vi "Parse Any Restric Data.vi"(8 "Error In":errorcluster, 10 "Data":string, 11 "ERD_Always Show in":T1) -> (0 "Error Out":errorcluster, 1 "CSV Data Out":string[](array[string]), 3 "ERD_Always Show out":T1)   [LabVIEW 2023]
uses:
  type defs/ERD_Always_Show_JL.ctl
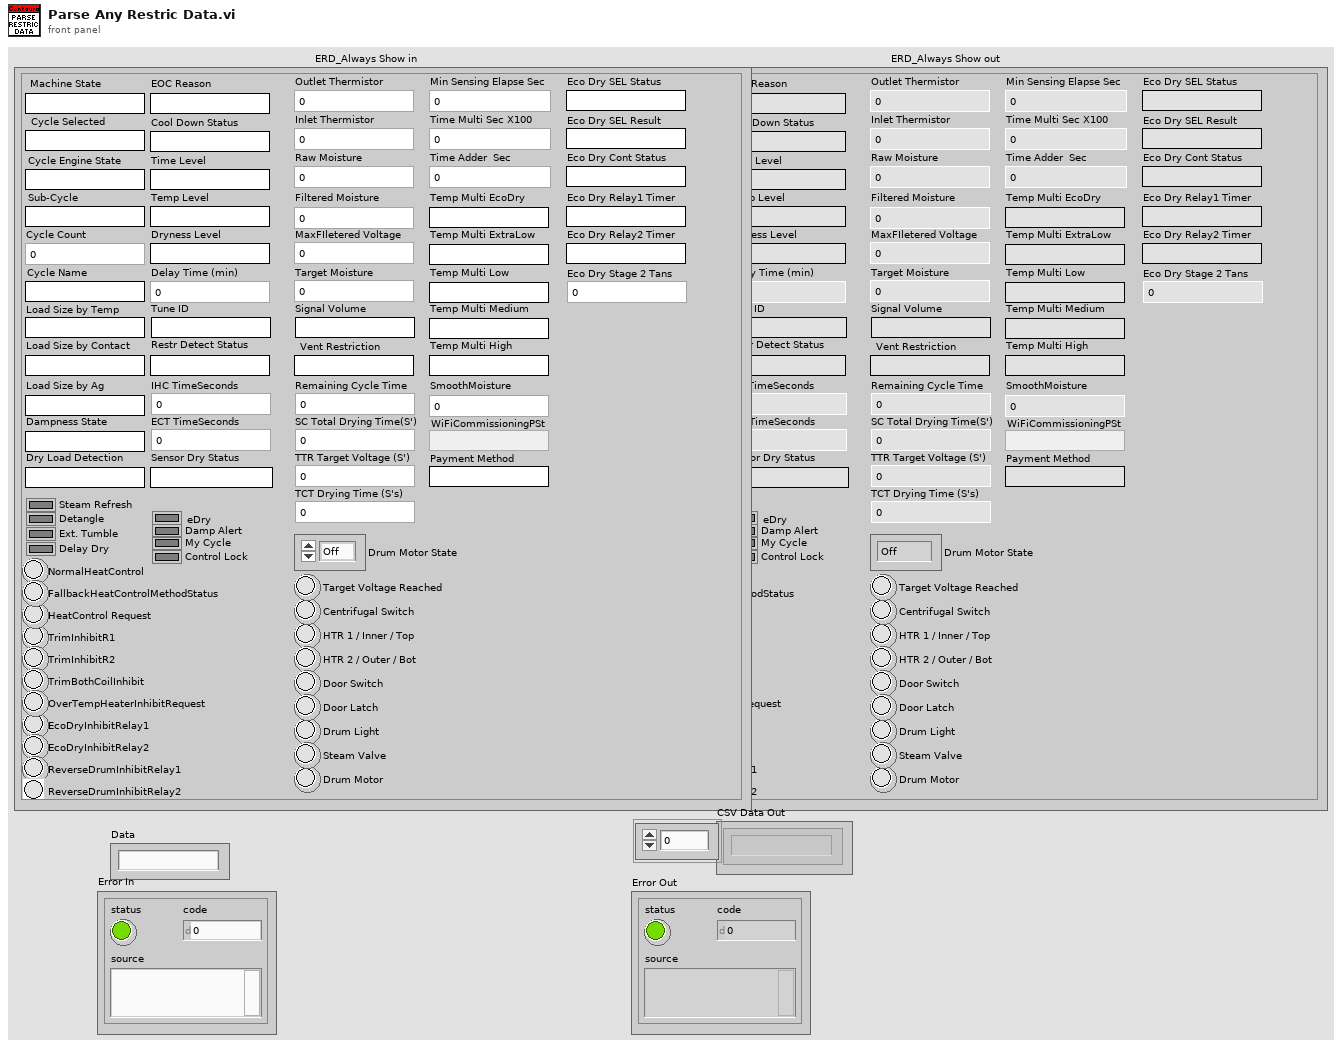
[diagram p1: front panel]
types:
  T1 = typedef "ERD_Always_Show_JL.ctl" = cluster{"Inlet Thermistor":u16, "Machine State":string, "Filtered Moisture":u16, "Cycle Selected":string, "HTR 1 / Inner / Top":bool, "HTR 2 / Outer / Bot":bool, "Door Switch":bool, "Drum Light":bool, "Cycle Engine State":string, "Centrifugal Switch":bool, "Drum Motor":bool, "Cycle Count":u32, "Ext. Tumble":bool, "eDry":bool, "Temp Level":string, "Dryness Level":string, "Time Level":string, "Delay Time (min)":u16, "Steam Refresh":bool, "Damp Alert":bool, "Sub-Cycle":string, "Outlet Thermistor":u16, "Target Moisture":u16, "Remaining Cycle Time":u32, "Raw Moisture":u16, "Cycle Name":string, "My Cycle":bool, "Delay Dry":bool, "Detangle":bool, "Control Lock":bool, "Steam Valve":bool, "Door Latch":bool, "Signal Volume":string, "Tune ID":string, "Restr Detect Status":string, "Vent Restriction":string, "Load Size by Contact":string, "Load Size by Temp":string, "EOC Reason":string, "Sensor Dry Status":string, "Dampness State":string, "Target Voltage Reached":bool, "TrimInhibitR1":bool, "TrimInhibitR2":bool, "TrimBothCoilInhibit":bool, "NormalHeatControl":bool, "HeatControl Request":bool, "Cool Down Status":string, "EcoDryInhibitRelay1":bool, "EcoDryInhibitRelay2":bool, "ReverseDrumInhibitRelay1":bool, "ReverseDrumInhibitRelay2":bool, "OverTempHeaterInhibitRequest":bool, "FallbackHeatControlMethodStatus":bool, "IHC TimeSeconds":u32, "ECT TimeSeconds ":u32, "SC Total Drying Time(S')":u32, "TTR Target Voltage (S')":u32, "TCT Drying Time (S's)":u32, "Drum Motor State":enum16{"Off", "Cw", "Ccw", "Max"}, "Load Size by Ag":string, "MaxFIletered Voltage":u16, "Dry Load Detection":string, "Min Sensing Elapse Sec":u32, "Time Multi Sec X100":u32, "Time Adder  Sec":u32, "Temp Multi EcoDry":string, "Temp Multi ExtraLow":string, "Temp Multi Low ":string, "Temp Multi Medium":string, "Temp Multi High":string, "SmoothMoisture":u16, "Eco Dry SEL Status":string, "Eco Dry SEL Result":string, "Eco Dry Cont Status":string, "Eco Dry Relay1 Timer":string, "Eco Dry Relay2 Timer ":string, "Eco Dry Stage 2 Tans ":u32, "WiFiCommissioningPSt":string, "Payment Method":string}
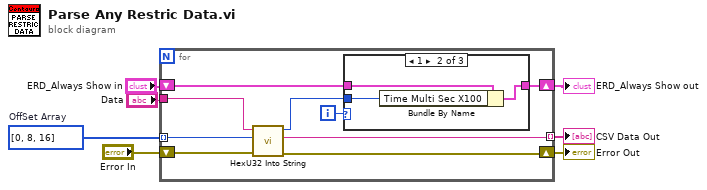
[diagram p0: block diagram]
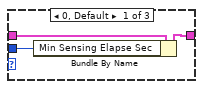
[diagram p2: hidden frame]
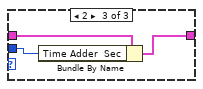
[diagram p3: hidden frame]
diagram:
  w2 = i32[] [0, 8, 16]  # OffSet Array
  n1 = for {
    tunnel: "Data" -> [w16]
    shift-right: [w12] -> w5
    shift-left: "ERD_Always Show in" -> [w13]
    tunnel: [w11] -> w4 mode=indexing
    shift-right: [w9] -> w1
    shift-left: "Error In" -> [w10]
    tunnel: w2 -> [w8] mode=indexing
    i -> [w15]
    n2 = call "HexU32 Into String.vi"("Error In"=w10, "offset (0)"=w8, "Input Data"=w16) -> ("Error Out"=w9:errorcluster, 2:"Parsed Number Out"=w11:string, 3:"Parsed Number Out"=w14:u32)  [unwired: 6 in]
    n3 = case shown="1" w15 {
      tunnel: w14 -> [w19 w22 w25]
      tunnel: w13 -> [w18 w21 w24]
      tunnel: [w17 w20 w23] -> w12
      frame 0, Default {
        n4 = Bundle By Name(cluster=w18, "Min Sensing Elapse Sec"=w19) -> (w17:T1)
      }
      frame 1 {
        n5 = Bundle By Name(cluster=w21, "Time Multi Sec X100"=w22) -> (w20:T1)
      }
      frame 2 {
        n6 = Bundle By Name(cluster=w24, "Time Adder  Sec"=w25) -> (w23:T1)
      }
    }
  }
  "ERD_Always Show out" <- w5
  "CSV Data Out" <- w4
  "Error Out" <- w1
